vi "Math-Compute Group Delay.vi"(0 "Frequency (Hz)":dbl[](array[numeric]), 5 "Phase (cycles)":dbl[](array[numeric]), 9 "Fmax (Hz)":dbl=inf) -> (4 "Group Delay (ms)":dbl, 8 "Intercept (cycles)":dbl)   [LabVIEW 2015]
uses:
  <vilib>/Analysis/NI_AALPro.lvlib
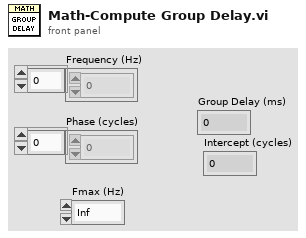
[diagram p1: front panel]
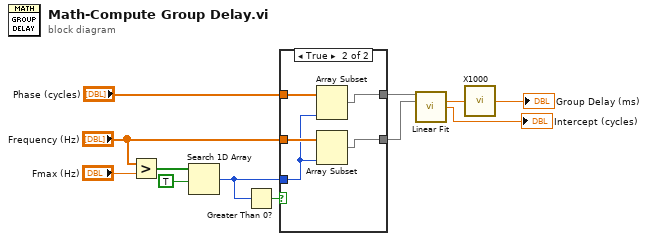
[diagram p0: block diagram]
diagram:
  n1 = Greater?(x="Frequency (Hz)", y="Fmax (Hz)") -> (0:w11:bool[])
  n2 = Search 1D Array(1D array=w11, element=TRUE) -> (index of element=w6:i32)  [unwired: 1 in]
  n3 = Greater Than 0?(x=w6) -> (x > 0?=w8:bool)
  n4 = case shown="True" w8 {
    tunnel: "Frequency (Hz)" -> [w14 w19]
    tunnel: [w14 w18] -> w5
    tunnel: "Phase (cycles)" -> [w13 w17]
    tunnel: [w13 w15] -> w4
    tunnel: w6 -> [_ w16]
    frame False {
    }
    frame True {
      n5 = Array Subset(array=w17, length=w16) -> (w15:dbl[])  [unwired: 1 in]
      n6 = Array Subset(array=w19, length=w16) -> (w18:dbl[])  [unwired: 1 in]
    }
  }
  n7 = call <vilib>:"Linear Fit.vi"("Y"=w4, "X"=w5) -> ("slope"=w3:dbl, "intercept"=→"Intercept (cycles)":dbl)  [unwired: 9 in, 3 out]
  n8 = call "X1000.vi"("X"=w3) -> ("X/1000"=→"Group Delay (ms)":dbl)
